vi "GetBookingList.vi"(8 "error in (no error)":errorcluster, 11 "ByteGSWebAPI-V0 in":refnum<class "ByteGSWebAPI-V0.lvclass">) -> (0 "error out":errorcluster, 2 "BookingList":T1[](array[typedef]), 3 "ByteGSWebAPI-V0 out":refnum<class "ByteGSWebAPI-V0.lvclass">)   [LabVIEW 2019, in "ByteGSWebAPI.lvlib" / "ByteGSWebAPI-V0.lvclass"]
doc: "Richiesta di GET di tutti i booking instruments (ID: \" \")"
uses:
  ByteGSWebAPI-V0.lvclass
  Cntrls/SingleBookingInstruments.ctl
  54c15d21-1fd3-4ea8-80e2-c69b0da6434b.vi
  <vilib>/JDP Science/JSONtext/JSON text to Variant.vi
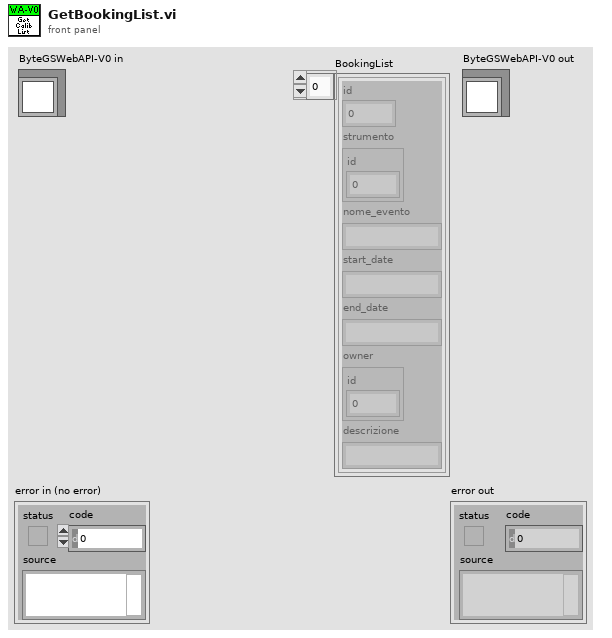
[diagram p1: front panel]
types:
  T1 = typedef "ByteGSWebAPI.lvlib/ByteGSWebAPI-V0.lvclass/SingleBookingInstruments.ctl" = cluster{"id":i32, "strumento":cluster{"id":i32}, "nome_evento":string, "start_date":string, "end_date":string, "owner":cluster{"id":i32}, "descrizione":string}
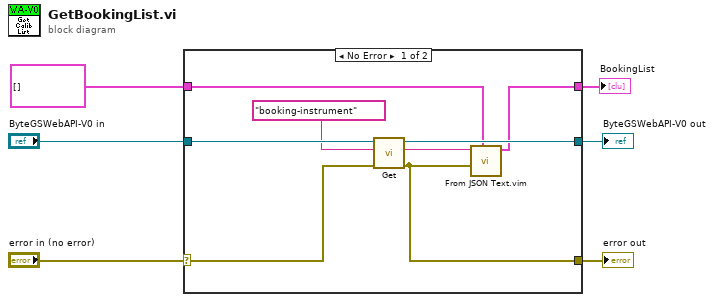
[diagram p0: block diagram]
diagram:
  n1 = case shown="No Error" "error in (no error)" {
    selector: "error in (no error)" -> [w11 w17]
    tunnel: [w7 w17] -> w5
    tunnel: [w13 w16] -> w3
    tunnel: "ByteGSWebAPI-V0 in" -> [w14 w16]
    tunnel: T1[] [] -> [w9 w15]
    tunnel: [w8 w15] -> w1
    frame No Error {
      n2 = call "Get.vi"("error in (no error)"=w11, "Request"="booking-instrument" ("Parameter"), "ByteGSWebAPI-V0 in"=w14) -> ("error out"=w7:errorcluster, "body"=w10:string, "ByteGSWebAPI-V0 out"=w13:refnum<class "ByteGSWebAPI-V0.lvclass">)  [unwired: 5 in, 1 out]
      n3 = call "From JSON Text.vim"("Data Type and Default Value"=w9, "error in (no error)"=w7, "JSON"=w10) -> ("Data out"=w8:T1[])  [unwired: 7 in, 1 out]
    }
    frame Error {
    }
  }
  "error out" <- w5
  "ByteGSWebAPI-V0 out" <- w3
  "BookingList" <- w1
